vi "LEP_RV_MapFileParser.vi"(0 "map file":path, 5 "error in (no error)":errorcluster) -> (12 "regions":T1(array[cluster])=[{"region name"="ER_IROM1", "size"=58800, "max"=262144, "contains heap?"=FALSE, "RAM?"=FALSE}, {"region name"="RW_IRAM1", "size"=41632, "max"=65536, "contains heap?"=TRUE, "RAM?"=FALSE}], 14 "total used ROM":u32, 15 "total available ROM":u32, 16 "total used RAM":u32, 17 "total available RAM":u32, 18 "heap size":i32, 19 "error out":errorcluster)   [LabVIEW 2011]
panel:
  out "total ROM size":i32=59016
  out "total RW size":i32=41632
  out "total RO size":i32=58800
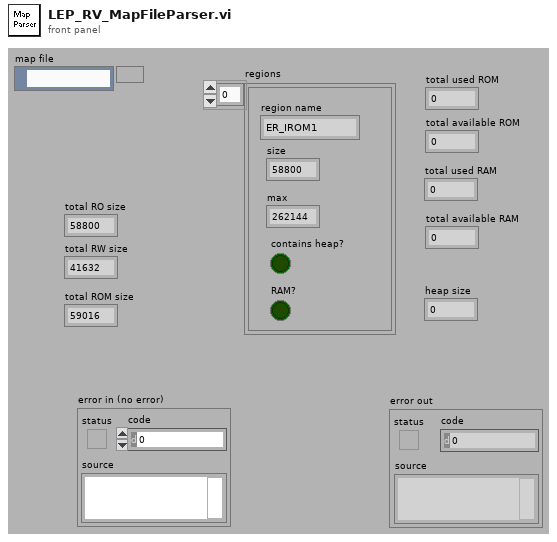
[diagram p1: front panel]
types:
  T1 = cluster{"region name":string, "size":u32, "max":u32, "contains heap?":bool, "RAM?":bool}[]
  T2 = cluster{"region name":string, "size":u32, "max":u32, "contains heap?":bool, "RAM?":bool}
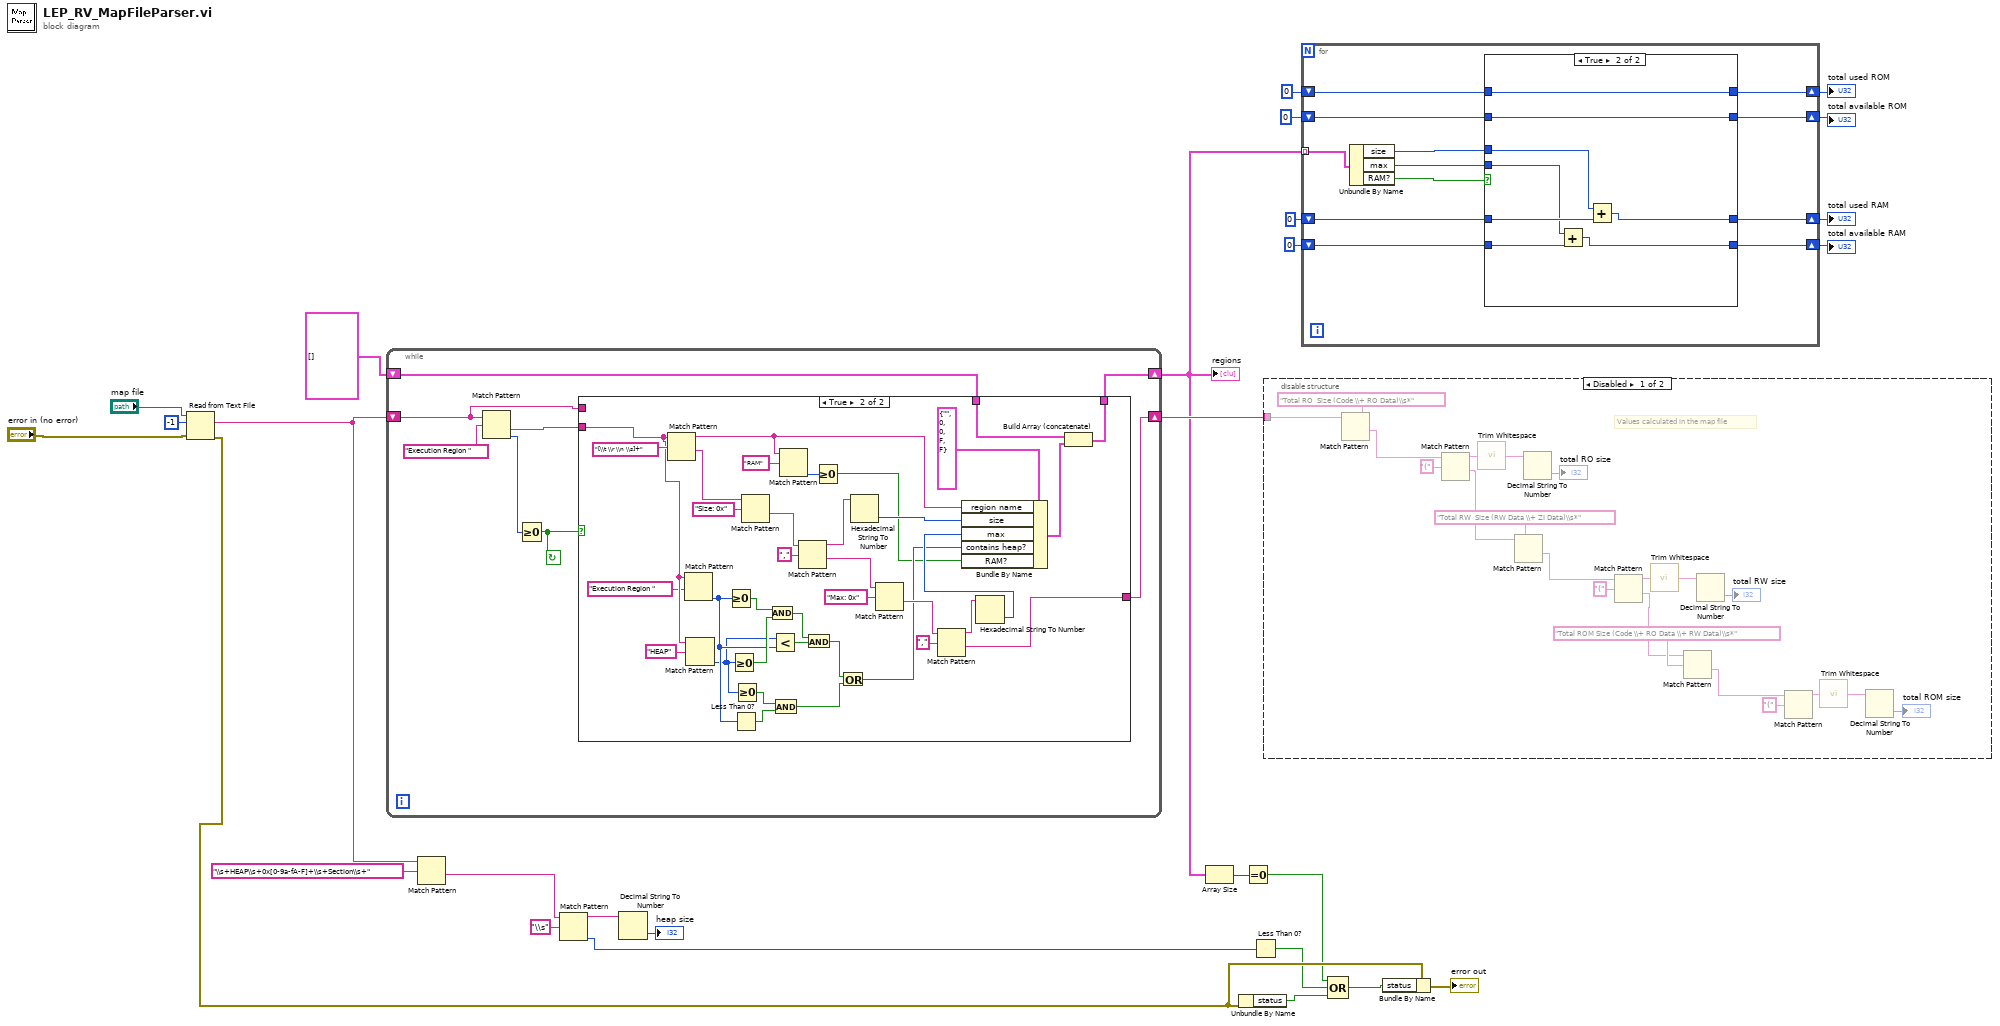
[diagram p0: block diagram]
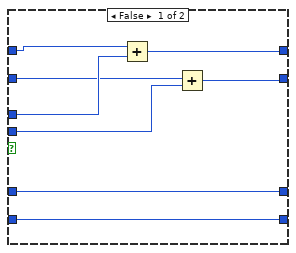
[diagram p2: hidden frame]
diagram:
  n1 = Read from Text File(file (use dialog)="map file", count=-1, error in="error in (no error)") -> (text=w20:string, error out=w6:errorcluster)  [unwired: 1 in, 2 out]
  n2 = while {
    shift-right: [w32] -> w27
    shift-left: w20 -> [w29]
    shift-right: [w30] -> w8
    shift-left: T1 [] ("regions 2") -> [w31]
    stop <- w33 continue-if-true
    n3 = Match Pattern(string=w29, regular expression="Execution Region ") -> (after substring=w35:string, offset past match=w34:i32)  [unwired: 1 in, 2 out]
    n4 = Greater Or Equal To 0?(x=w34) -> (x >= 0?=w33:bool)
    n5 = case shown="True" w33 {
      tunnel: w35 -> [_ w57]
      tunnel: [w37 w63] -> w32
      tunnel: w31 -> [w38 w60]
      tunnel: [w38 w58] -> w30
      tunnel: w29 -> [w37 _]
      frame False {
      }
      frame True {
        n6 = Match Pattern(string=w57, regular expression="[\\t \\r \\n \\s]+") -> (before substring=w42:string, after substring=w73:string)  [unwired: 1 in, 2 out]
        n7 = Match Pattern(string=w57, regular expression="Execution Region ") -> (offset past match=w50:i32)  [unwired: 1 in, 3 out]
        n8 = Match Pattern(string=w57, regular expression="HEAP") -> (offset past match=w49:i32)  [unwired: 1 in, 3 out]
        n9 = Greater Or Equal To 0?(x=w50) -> (x >= 0?=w54:bool)
        n10 = Greater Or Equal To 0?(x=w49) -> (x >= 0?=w53:bool)
        n11 = Less Than 0?(x=w50) -> (x < 0?=w47:bool)
        n12 = Greater Or Equal To 0?(x=w49) -> (x >= 0?=w48:bool)
        n13 = Match Pattern(string=w73, regular expression="Size: 0x") -> (after substring=w70:string)  [unwired: 1 in, 3 out]
        n14 = And(x=w54, y=w53) -> (x .and. y?=w52:bool)
        n15 = Less?(x=w49, y=w50) -> (x < y?=w51:bool)
        n16 = And(x=w48, y=w47) -> (x .and. y?=w45:bool)
        n17 = Match Pattern(string=w42, regular expression="RAM") -> (offset past match=w40:i32)  [unwired: 1 in, 3 out]
        n18 = Match Pattern(string=w70, regular expression=",") -> (before substring=w65:string, after substring=w66:string)  [unwired: 1 in, 2 out]
        n19 = And(x=w52, y=w51) -> (x .and. y?=w46:bool)
        n20 = Greater Or Equal To 0?(x=w40) -> (x >= 0?=w39:bool)
        n21 = Or(x=w46, y=w45) -> (x .or. y?=w44:bool)
        n22 = Hexadecimal String To Number(string=w65) -> (number=w62:u32)  [unwired: 2 in, 1 out]
        n23 = Match Pattern(string=w66, regular expression="Max: 0x") -> (after substring=w69:string)  [unwired: 1 in, 3 out]
        n24 = Match Pattern(string=w69, regular expression=",") -> (before substring=w64:string, after substring=w63:string)  [unwired: 1 in, 2 out]
        n25 = Hexadecimal String To Number(string=w64) -> (number=w61:u32)  [unwired: 2 in, 1 out]
        n26 = Bundle By Name(cluster=T2 {"region name"="", "size"=0, "max"=0, "contains heap?"=FALSE, "RAM?"=FALSE} ("region"), "region name"=w42, "size"=w62, "max"=w61, "contains heap?"=w44, "RAM?"=w39) -> (w59:T2)
        n27 = Build Array (concatenate)(w60, w59) -> (w58:T1)
      }
    }
  }
  "regions" <- w8
  n28 = Match Pattern(string=w20, regular expression="\\s+HEAP\\s+0x[0-9a-fA-F]+\\s+Section\\s+") -> (after substring=w24:string)  [unwired: 1 in, 3 out]
  n29 = Match Pattern(string=w24, regular expression="\\s") -> (before substring=w23:string, offset past match=w9:i32)  [unwired: 1 in, 2 out]
  n30 = Decimal String To Number(string=w23) -> (number=→"heap size":i32)  [unwired: 2 in, 1 out]
  n31 = Array Size(array=w8) -> (size(s)=w7:i32)
  n32 = Unbundle By Name(w6) -> ("status"=w2:bool)
  n33 = Equal To 0?(x=w7) -> (x = 0?=w3:bool)
  n34 = Less Than 0?(x=w9) -> (x < 0?=w4:bool)
  n35 = disable-structure shown="Disabled" {
    disable-tunnel: w27 -> [w95 _]
    frame Disabled {
      # "Values calculated in the map file"
      n36 = Match Pattern(string=w95, regular expression="Total RO  Size (Code \\+ RO Data)\\s*") -> (after substring=w93:string)  [unwired: 1 in, 3 out]
      n37 = Match Pattern(string=w93, regular expression="(") -> (before substring=w91:string, after substring=w76:string)  [unwired: 1 in, 2 out]
      n38 = call <vilib>:"Trim Whitespace.vi"("string"=w91) -> ("trimmed string"=w90:string)  [unwired: 1 in]
      n39 = Match Pattern(string=w76, regular expression="Total RW  Size (RW Data \\+ ZI Data)\\s*") -> (after substring=w84:string)  [unwired: 1 in, 3 out]
      n40 = Decimal String To Number(string=w90) -> (number=→"total RO size":i32)  [unwired: 2 in, 1 out]
      n41 = Match Pattern(string=w84, regular expression="(") -> (before substring=w86:string, after substring=w75:string)  [unwired: 1 in, 2 out]
      n42 = call <vilib>:"Trim Whitespace.vi"("string"=w86) -> ("trimmed string"=w87:string)  [unwired: 1 in]
      n43 = Match Pattern(string=w75, regular expression="Total ROM Size (Code \\+ RO Data \\+ RW Data)\\s*") -> (after substring=w81:string)  [unwired: 1 in, 3 out]
      n44 = Decimal String To Number(string=w87) -> (number=→"total RW size":i32)  [unwired: 2 in, 1 out]
      n45 = Match Pattern(string=w81, regular expression="(") -> (before substring=w79:string)  [unwired: 1 in, 3 out]
      n46 = call <vilib>:"Trim Whitespace.vi"("string"=w79) -> ("trimmed string"=w78:string)  [unwired: 1 in]
      n47 = Decimal String To Number(string=w78) -> (number=→"total ROM size":i32)  [unwired: 2 in, 1 out]
    }
    frame Enabled {
    }
  }
  n48 = for {
    tunnel: w8 -> [w107] mode=indexing
    shift-right: [w99] -> w15
    shift-left: u32 0 ("size") -> [w101]
    shift-right: [w98] -> w14
    shift-left: u32 0 ("size") -> [w100]
    shift-right: [w96] -> w13
    shift-left: u32 0 ("size") -> [w103]
    shift-right: [w97] -> w12
    shift-left: u32 0 ("size") -> [w102]
    n49 = Unbundle By Name(w107) -> ("size"=w105:u32, "max"=w104:u32, "RAM?"=w106:bool)
    n50 = case shown="True" w106 {
      tunnel: w105 -> [w113 w118]
      tunnel: w104 -> [w112 w119]
      tunnel: w103 -> [w115 w121]
      tunnel: w102 -> [w114 w120]
      tunnel: w101 -> [w110 w123]
      tunnel: w100 -> [w111 w122]
      tunnel: [w108 w123] -> w99
      tunnel: [w109 w122] -> w98
      tunnel: [w114 w117] -> w97
      tunnel: [w115 w116] -> w96
      frame False {
        n51 = Add(x=w110, y=w113) -> (x+y=w108:u32)
        n52 = Add(x=w111, y=w112) -> (x+y=w109:u32)
      }
      frame True {
        n53 = Add(x=w119, y=w120) -> (x+y=w117:u32)
        n54 = Add(x=w118, y=w121) -> (x+y=w116:u32)
      }
    }
  }
  "total used ROM" <- w15
  "total available ROM" <- w14
  "total used RAM" <- w13
  "total available RAM" <- w12
  n55 = Compound Arithmetic op=OR(w3, w4, w2) -> (w1:bool)
  n56 = Bundle By Name(cluster=w6, "status"=w1) -> (→"error out":errorcluster)
